vi "PROJEKAT RUKE-final.vi"() -> ()   [LabVIEW 2014]
doc: "This example shows a robotic arm with four revolute joints (a 4R serial robot), and demonstrates how to use custom equations to deterministically compute inverse kinematics for the arm."
uses:
  <vilib>/Analysis/Matrix/Datatypes/RealMatrix.ctl
  <vilib>/Platform/TimedLoop/XDataNode/timing_clust.ctl
  <vilib>/Platform/TimedLoop/XDataNode/nitl_modes.ctl
  <vilib>/Platform/TimedLoop/XDataNode/wakeup.ctl
  <vilib>/robotics/Kinematics/Plotting/Tree Element.ctl
  <vilib>/robotics/Kinematics/Plotting/Element Type.ctl
  <vilib>/robotics/Kinematics/Plotting/Joint Type.ctl
  Projekat SNJ+ED/Timer 2013/Control Timer.ctl
  <vilib>/Utility/inputDevices.llb/joystickAcquire.vi
  <vilib>/Analysis/Matrix/Numeric/Multiply/Multiply - R,RM.vi
  <vilib>/Analysis/Matrix/Numeric/Add/Add - RM,RM.vi
  <vilib>/Analysis/Matrix/Numeric/Multiply/Multiply - RM,R.vi
  <vilib>/NXT/Dual Mode Library/prims/inRangeAndCoerce/inRangeAndCoerce_float.vi
  <vilib>/addons/Fuzzy Logic/FL Fuzzy Controller (MISO).vi
  <vilib>/picture/3D Picture Control/Object/Create Object (name).vi
  <vilib>/picture/3D Picture Control/Helpers/Apply Texture (no reference).vi
  <vilib>/picture/3D Picture Control/Object/Add Object (no reference).vi
  <vilib>/Utility/inputDevices.llb/closeJoystick.vi
  <vilib>/platform/TimedLoop/XDataNode/XDataNode.xnode
  <vilib>/robotics/Kinematics/Plotting/NI_Robotics_3DKinematics.lvlib
  <vilib>/Analysis/Matrix/NI_Matrix.lvlib
  <vilib>/Platform/TimedLoop/XDataNode/XDNodeRunTimeDep.lvlib
  <vilib>/addons/Fuzzy Logic/NI_Fuzzy_Logic_API.lvlib
  <vilib>/picture/3D Picture Control/NI_3D Picture Control.lvlib
panel:
  in  "square":bool
  in  "Triangle":bool
  out "UDP Y":dbl(graph)
  out "UDP X":dbl(graph)
  out "UDP Y":dbl
  out "UDP X":dbl
  in  "Enum":T1(ring)
  out "output boosted":dbl
  out "fuzzy 1":dbl=-0.3643519039326156
  out "output":dbl=0.0001328998348474089
  in  "Kp2":dbl=120.0
  in  "Ki2":dbl=0.0005
  in  "Kd2":dbl=3.0
  in  "fuzzy za joint 2":bool=TRUE
  out "Fuzzy Kp":dbl=600.1063198678779
  in  "SMC J2":dbl=23.0
  in  "fuzzy za joint 1":bool=TRUE
  in  "Kp1":dbl=700.0
  out "Ycontroller":dbl
  out "Xcontroller":dbl
  in  "SMC J1":dbl=23.0
  in  "PID":bool=TRUE
  in  "stanja":T2
  in  "circle":bool
  in  "Kd1":dbl=20.0
  in  "Ki1":dbl=0.01
  out "error joint 2":dbl=0.8817520547054016
  out "error joint 1":dbl=-1.5374954740064481
  in  "Joint angles requested":dbl[](array[numeric])=[0.0, -2.3551534008356274, 2.0586714743351897, 0.0]
  out "Torque 2":sgl(graph)=9.405421
  out "Torque 1":sgl(graph)=-10.80559
  out "axis 2":cluster{"Joint Angles":dbl, "Joint Angles":dbl}(graph)={"Joint Angles"=117.07143482867573, "Joint Angles"=117.95318688338114}
  out "axis 1":cluster{"Joint Angles":dbl, "Joint Angles":dbl}(graph)={"Joint Angles"=-133.40285449975764, "Joint Angles"=-134.94034997376409}
  out "T requested":T3=[[-10.805589299068552], [9.40542142349445]]
  out "Qenc":T3=[[-2.3283250726964995], [2.0432778992607856]]
  out "dQenc":T3=[[-0.00014660765716752367], [-8.377580409572782e-05]]
  in  "enc resolution":dbl=900000.0
  out "dQ":T3=[[-0.0001628688682452542], [-6.482032013744222e-05]]
  out "Q":T3=[[-2.3283199705917617], [2.043281569449471]]
  out "T":T3=[[-10.80558967590332], [9.405421257019043]]
  in  "Y":dbl(slide)=-1.0 scale=-1.0..1.0
  in  "X":dbl(slide)=0.24999999999999994 scale=-1.5..1.5
  in  "actutator max torque":sgl(slide)=100.0 scale=0.0..100.0
  out "first overload":bool
  out "second overload":bool
  in  "controller on":bool=TRUE
  in  "Joint angles":dbl[](array[numeric])=[3.14, -2.3283199705917617, 2.043281569449471, 0.0]
  in  "stop":bool
  out "3D robotic arm":refnum<vi>(3d-picture)
  # "!!!VAZNO!!!\nPRE  POKRETANJA \n-POSTAVITI U TASK MANAGERU PRIORITET U REAL TIME\n-POKRENUTI PROJEKAT PA GA STOPIRATI I PONOVO POKRENUTI"
  # "Naèini kontrole"
  # "UDP za computer vision"
  # "HID uredjaj"
  # "Predefinisane putanje"
  # "Strategije upravljanja"
  # "PID parametri"
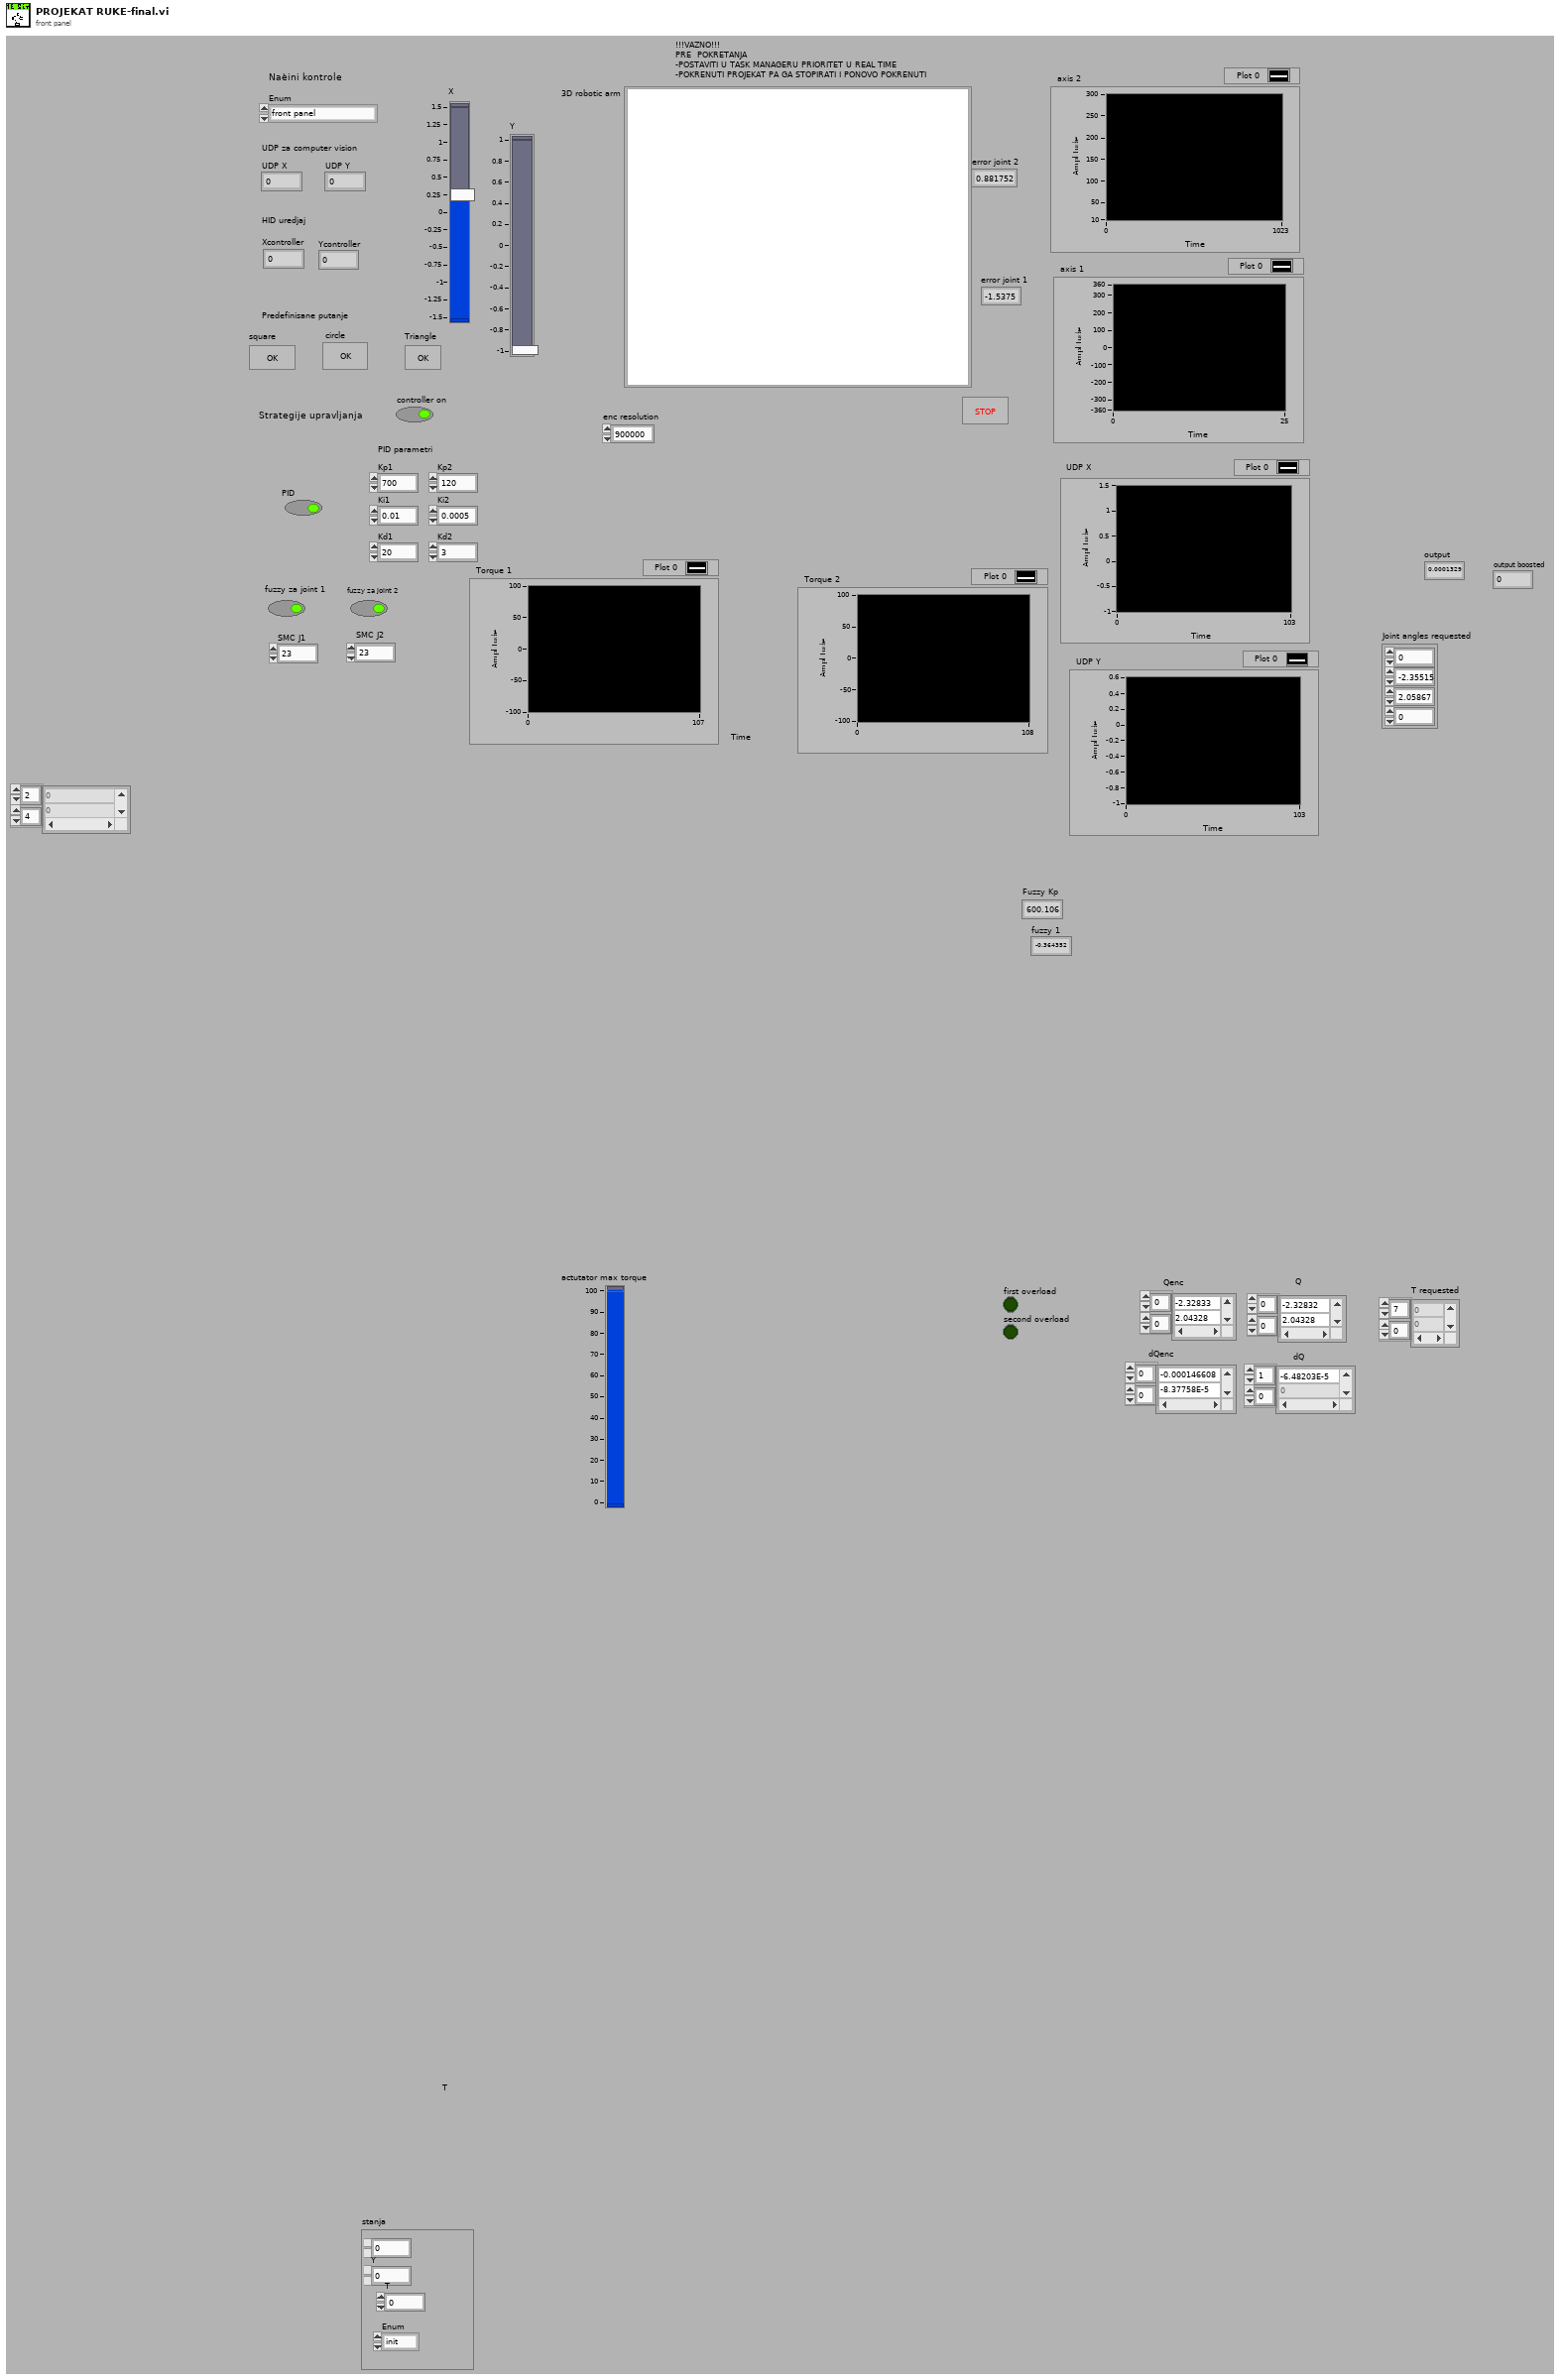
[diagram p1: front panel]
types:
  T1 = enum16{"front panel", "producer consumer", "hid", "udp"}
  T2 = cluster{"X":dbl, "Y":dbl, "T":dbl, "Enum":enum16{"init", "wait", "execute", "shutdown"}}
  T3 = typedef "NI_Matrix.lvlib/RealMatrix.ctl" = dbl[][]
  T4 = cluster{"Red":sgl, "Green":sgl, "Blue":sgl, "Alpha":sgl}
  T5 = typedef "NI_Robotics_3DKinematics.lvlib/Tree Element.ctl" = cluster{"Name":string, "Parent":string, "Type":T6, "Visible?":bool, "Geometry Definition":dbl[], "Position WRT Parent (X,Y,Z)":dbl[], "Rotation WRT Parent (degrees)":dbl[], "Joint Type":T7, "Geometry File Path":path, "Indent Level":i32, "Color":u32}
  T6 = typedef "NI_Robotics_3DKinematics.lvlib/Element Type.ctl" = enum16{"Joint", "Box", "Cylinder", "Cone", "Sphere", "ASE File", "VRML File", "STL File", "Space"}
  T7 = typedef "NI_Robotics_3DKinematics.lvlib/Joint Type.ctl" = enum16{"Trans_X", "Trans_Y", "Trans_Z", "Rot_X", "Rot_Y", "Rot_Z", "None"}
  T8 = typedef "NI_Fuzzy_Logic_API.lvlib/FL System.ctl" = cluster{"input variables":T9[], "output variables":T9[], "rules":T12[], "defuzzification method":T18, "description":string, "user MF interpolating polynomials":T19[]}
  T9 = typedef "NI_Fuzzy_Logic_API.lvlib/FL Variable.ctl" = cluster{"name":string, "range":dbl[], "MFs":T10[]}
  T10 = typedef "NI_Fuzzy_Logic_API.lvlib/FL Membership Function.ctl" = cluster{"name":string, "shape":T11, "points":dbl[], "color":u32, "user-defined shape index":i32}
  T11 = typedef "NI_Fuzzy_Logic_API.lvlib/FL Membership Function Shape.ctl" = u16
  T12 = typedef "NI_Fuzzy_Logic_API.lvlib/FL Rule.ctl" = cluster{"antecedents":T13[], "antecedent connective":T15, "consequents":T16[], "consequent implication":T17, "degree of support":dbl}
  T13 = typedef "NI_Fuzzy_Logic_API.lvlib/FL Antecedent.ctl" = cluster{"Var Index":i32, "MF Index":i32, "Cond":T14}
  T14 = typedef "NI_Fuzzy_Logic_API.lvlib/FL Modifier.ctl" = u16
  T15 = typedef "NI_Fuzzy_Logic_API.lvlib/FL Antecedent Connective.ctl" = u16
  T16 = typedef "NI_Fuzzy_Logic_API.lvlib/FL Consequent.ctl" = cluster{"Var Index":i32, "MF Index":i32, "Cond":T14}
  T17 = typedef "NI_Fuzzy_Logic_API.lvlib/FL Consequent Implication.ctl" = u16
  T18 = typedef "NI_Fuzzy_Logic_API.lvlib/FL Defuzzification.ctl" = u16
  T19 = typedef "NI_Fuzzy_Logic_API.lvlib/FL Interpolating polynomials.ctl" = cluster{"X":dbl[], "Y":dbl[], "Y(x) coeff":dbl[][], "X(y) coeff":dbl[][], "Area(y) coeff":dbl[][], "coa_x(y) coeff":dbl[][]}
  T20 = typedef "XDNodeRunTimeDep.lvlib/timing_clust.ctl" = cluster{"Expected End [f-1]":u64, "Actual End [f-1]":u64, "Finished Late? [f-1]":bool, "Expected End [i-1]":u64, "Actual End [i-1]":u64, "Finished Late? [i-1]":bool, "Expected Start [i]":u64, "Actual Start [i]":u64, "Expected Start [f]":u64, "Actual Start [f]":u64, "Source Name":string, "Structure Name":string, "Period":i64, "Deadline":i64, "Offset":i64, "Start":i64, "Priority":i32, "Timeout":i32, "Mode":T21, "Wakeup Reason":T22, "Error":errorcluster, "Source Type":string, "Secondary Source Type":string, "Global End Time":u64, "Global Start Time":u64, "Frame Duration":u64, "Iteration Duration":u64, "Assigned CPU":i32, "I/O Scan Engine Mode":u32}
  T21 = typedef "XDNodeRunTimeDep.lvlib/nitl_modes.ctl" = enum32{"No Change", "Process missed periods, maintain original phase", "Discard missed periods, maintain original phase", "Process missed periods, ignore original phase", "Discard missed periods, ignore original phase"}
  T22 = typedef "XDNodeRunTimeDep.lvlib/wakeup.ctl" = enum32{"Normal", "Aborted", "Asynchronous wakeup", "Timing source error", "Timed loop error", "Timeout"}
  T23 = typedef "NI_Robotics_3DKinematics.lvlib/Joint Control.ctl" = cluster{"Joint Refnum":refnum<vi>, "Joint Type":T7, "Position WRT Parent":dbl[], "Rotation WRT Parent":dbl[], "Bar Refnum":refnum<vi>}
  T24 = typedef "Control Timer.ctl" = enum16{"Timecheck", "Reset"}
  T25 = typedef "imagedata.ctl" = cluster{"image type":i32, "image depth":i32, "image":u8[], "mask":u8[], "colors":u32[], "Rectangle":cluster{"left":i16, "top":i16, "right":i16, "bottom":i16}}
  T26 = cluster{"X":dbl, "Y":dbl, "T":dbl, "Enum":enum16{"init", "wait", "execute", "shutdown"}}[]
  T27 = cluster{"X axis":i32, "Y axis":i32, "Z axis":i32, "X axis rotation":i32, "Y axis rotation":i32, "Z axis rotation":i32, "U axis":i32, "V axis":i32}
  T28 = cluster{"button 1":bool, "button 2":bool, "button 3":bool, "button 4":bool, "button 5":bool, "button 6":bool, "button 7":bool, "button 8":bool, "button 9":bool, "button 10":bool, "button 11":bool, "button 12":bool, "button 13":bool, "button 14":bool, "button 15":bool, "button 16":bool, "button 17":bool, "button 18":bool, "button 19":bool, "button 20":bool, "button 21":bool, "button 22":bool, "button 23":bool, "button 24":bool, "button 25":bool, "button 26":bool, "button 27":bool, "button 28":bool, "button 29":bool, "button 30":bool, "button 31":bool, "button 32":bool}
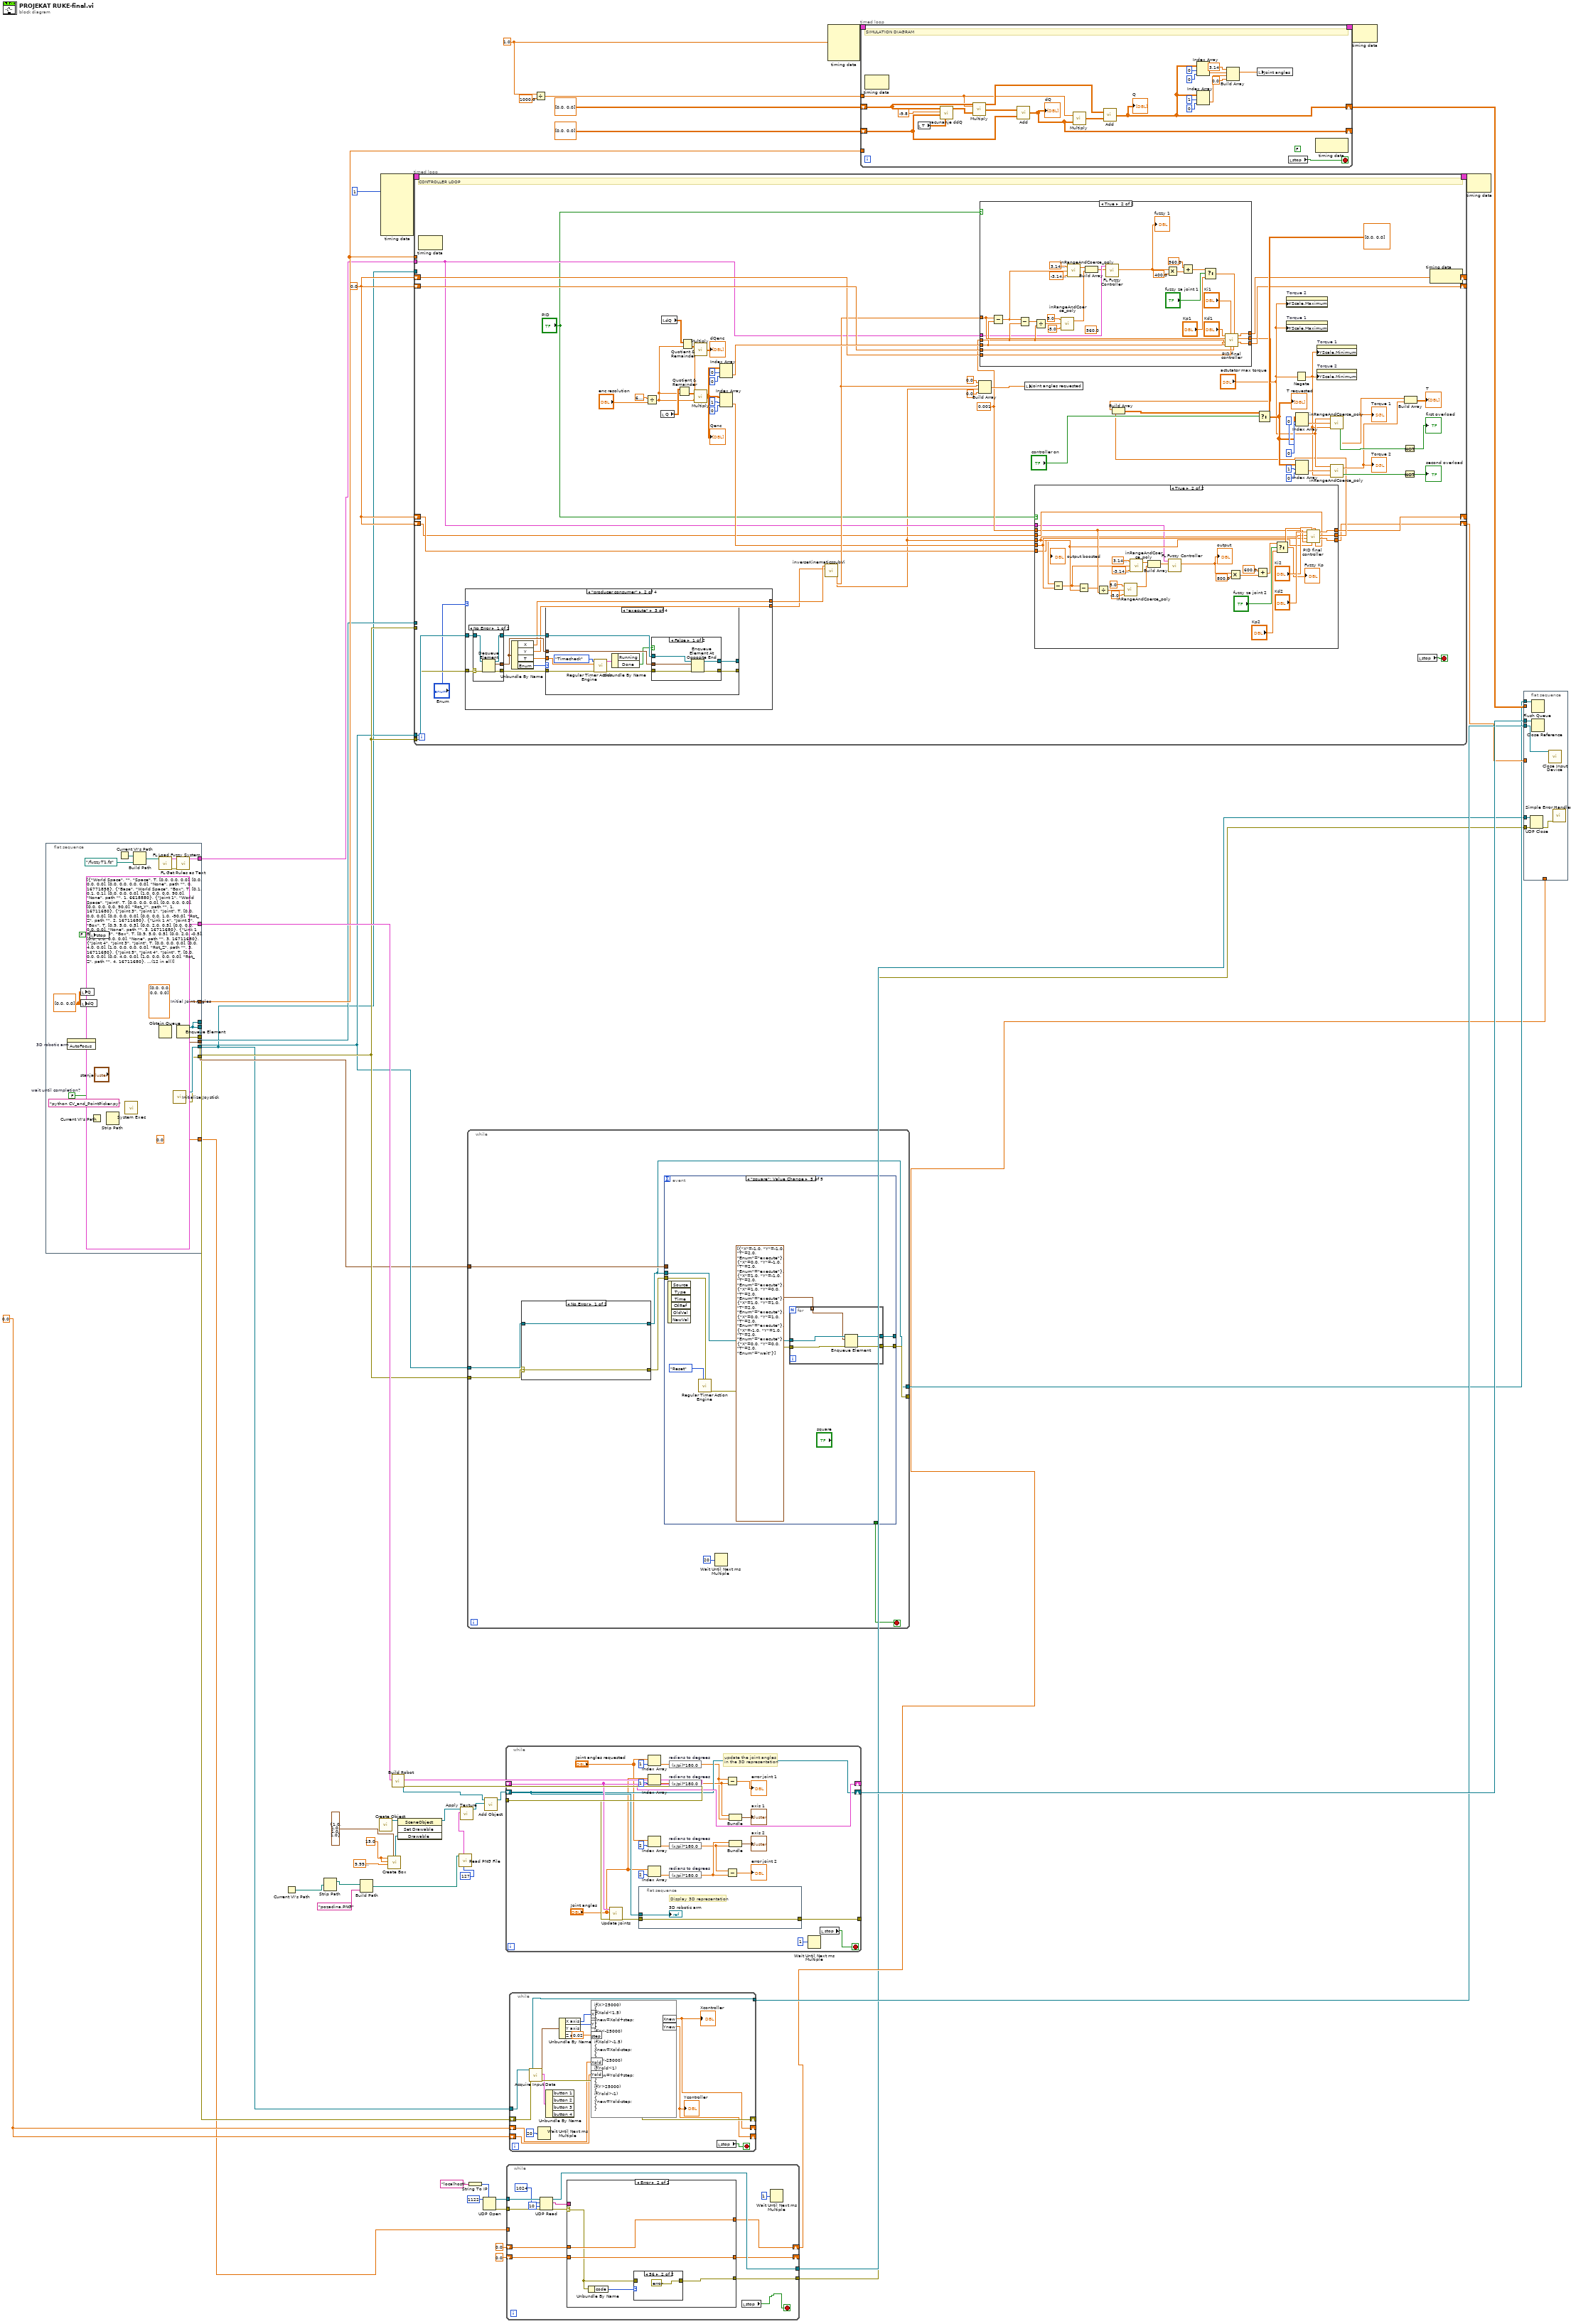
[diagram p0: block diagram]
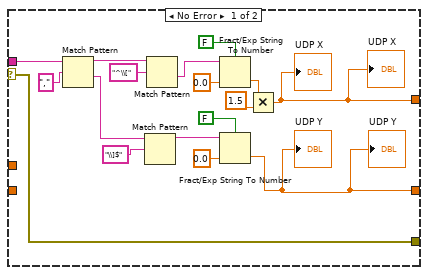
[diagram p2: hidden frame]
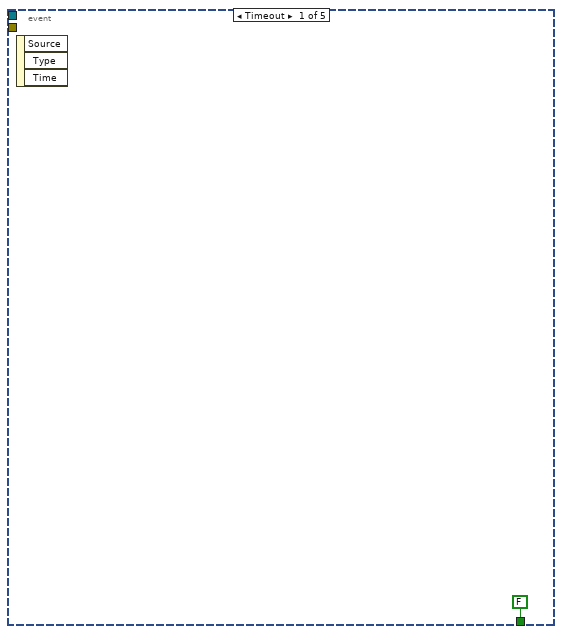
[diagram p4: hidden frame]
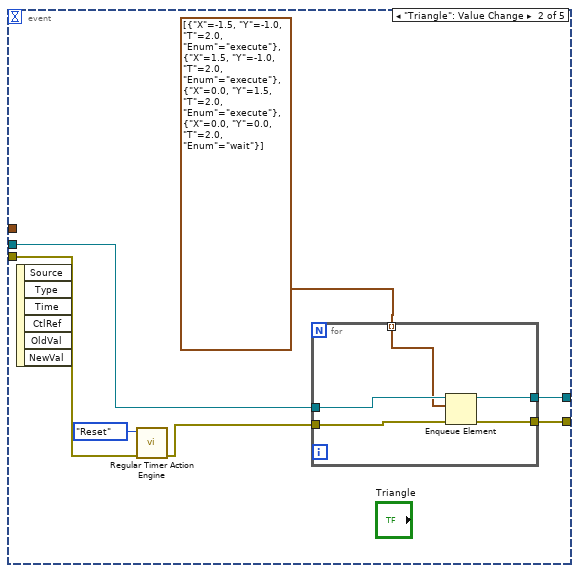
[diagram p5: hidden frame]
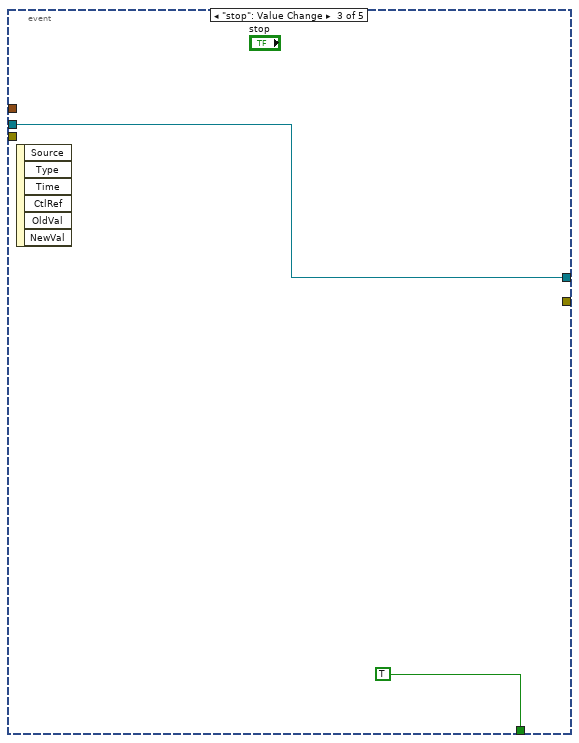
[diagram p6: hidden frame]
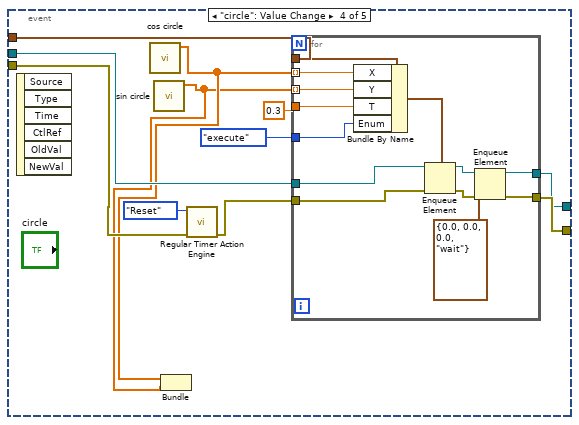
[diagram p7: hidden frame]
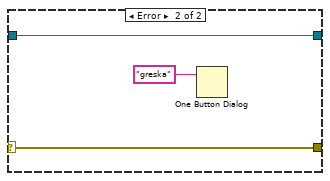
[diagram p8: hidden frame]
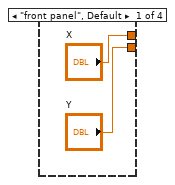
[diagram p9: hidden frame]
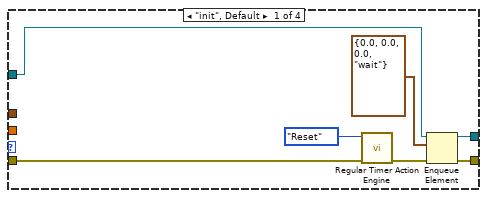
[diagram p10: hidden frame]
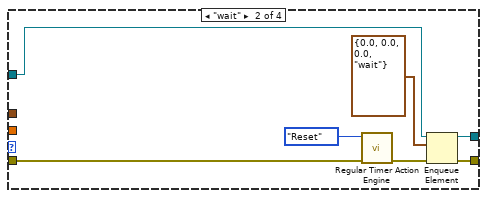
[diagram p11: hidden frame]
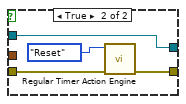
[diagram p12: hidden frame]
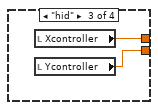
[diagram p15: hidden frame]
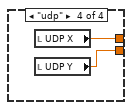
[diagram p16: hidden frame]
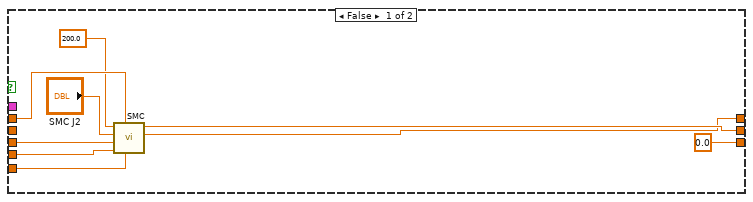
[diagram p17: hidden frame]
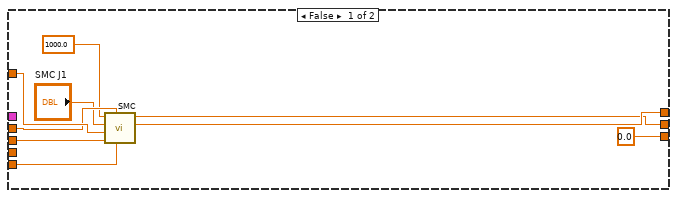
[diagram p18: hidden frame]
diagram:
  w23 = 0.0
  w26 = sgl 15.0 ("Length X")
  w38 = 0.0
  w39 = 1.0 ("simulation precision")
  n1 = flat-sequence {
    tunnel: [w76] -> w42
    tunnel: [T5[] [{"Name"="World Space", "Parent"="", "Type"=enum."Space", "Visible?"=TRUE, "Geometry Definition"=[0.0, 0.0, 0.0], "Position WRT Parent (X,Y,Z)"=[0.0, 0.0, 0.0], "Rotation WRT Parent (degrees)"=[0.0, 0.0, 0.0, 0.0], "Joint Type"=enum."None", "Geometry File Path"=path "", "Indent Level"=0, "Color"=16771858}, {"Name"="Base", "Parent"="World Space", "Type"=enum."Box", "Visible?"=TRUE, "Geometry Definition"=[0.1, 0.1, 0.1], "Position WRT Parent (X,Y,Z)"=[0.0, 0.0, 0.0], "Rotation WRT Parent (degrees)"=[1.0, 0.0, 0.0, 90.0], "Joint Type"=enum."None", "Geometry File Path"=path "", "Indent Level"=1, "Color"=6618880}, {"Name"="Joint 1", "Parent"="World Space", "Type"=enum."Joint", "Visible?"=TRUE, "Geometry Definition"=[0.0, 0.0, 0.0], "Position WRT Parent (X,Y,Z)"=[0.0, 0.0, 0.0], "Rotation WRT Parent (degrees)"=[0.0, 0.0, 0.0, 90.0], "Joint Type"=enum."Rot_Y", "Geometry File Path"=path "", "Indent Level"=1, "Color"=16711680}, {"Name"="Joint 3", "Parent"="Joint 1", "Type"=enum."Joint", "Visible?"=TRUE, "Geometry Definition"=[0.0, 0.0, 0.0], "Position WRT Parent (X,Y,Z)"=[0.0, 0.0, 0.0], "Rotation WRT Parent (degrees)"=[0.0, 0.0, 1.0, -90.0], "Joint Type"=enum."Rot_Z", "Geometry File Path"=path "", "Indent Level"=2, "Color"=16711680}, {"Name"="Link 1 A", "Parent"="Joint 3", "Type"=enum."Box", "Visible?"=TRUE, "Geometry Definition"=[0.9, 5.0, 0.5], "Position WRT Parent (X,Y,Z)"=[0.0, 2.0, 0.5], "Rotation WRT Parent (degrees)"=[0.0, 0.0, 0.0, 0.0], "Joint Type"=enum."None", "Geometry File Path"=path "", "Indent Level"=3, "Color"=16711680}, {"Name"="Link 1 B", "Parent"="Joint 3", "Type"=enum."Box", "Visible?"=TRUE, "Geometry Definition"=[0.9, 5.0, 0.5], "Position WRT Parent (X,Y,Z)"=[0.0, 2.0, -0.5], "Rotation WRT Parent (degrees)"=[0.0, 0.0, 0.0, 0.0], "Joint Type"=enum."None", "Geometry File Path"=path "", "Indent Level"=3, "Color"=16711680}, {"Name"="Joint 4", "Parent"="Joint 3", "Type"=enum."Joint", "Visible?"=TRUE, "Geometry Definition"=[0.0, 0.0, 0.0], "Position WRT Parent (X,Y,Z)"=[0.0, 4.0, 0.0], "Rotation WRT Parent (degrees)"=[1.0, 0.0, 0.0, 0.0], "Joint Type"=enum."Rot_Z", "Geometry File Path"=path "", "Indent Level"=3, "Color"=16711680}, {"Name"="Joint 5", "Parent"="Joint 4", "Type"=enum."Joint", "Visible?"=TRUE, "Geometry Definition"=[0.0, 0.0, 0.0], "Position WRT Parent (X,Y,Z)"=[0.0, 4.0, 0.0], "Rotation WRT Parent (degrees)"=[1.0, 0.0, 0.0, 0.0], "Joint Type"=enum."Rot_Z", "Geometry File Path"=path "", "Indent Level"=4, "Color"=16711680}, {"Name"="Lower Arm 1", "Parent"="Joint 4", "Type"=enum."Box", "Visible?"=TRUE, "Geometry Definition"=[0.9, 4.5, 0.5], "Position WRT Parent (X,Y,Z)"=[0.0, 1.75, 0.5], "Rotation WRT Parent (degrees)"=[0.0, 0.0, 0.0, 0.0], "Joint Type"=enum."None", "Geometry File Path"=path "", "Indent Level"=5, "Color"=16860}, {"Name"="Lower Arm 2", "Parent"="Joint 4", "Type"=enum."Box", "Visible?"=TRUE, "Geometry Definition"=[0.9, 4.5, 0.5], "Position WRT Parent (X,Y,Z)"=[0.0, 1.75, -0.5], "Rotation WRT Parent (degrees)"=[0.0, 0.0, 0.0, 0.0], "Joint Type"=enum."None", "Geometry File Path"=path "", "Indent Level"=5, "Color"=16860}, {"Name"="Hand", "Parent"="Joint 4", "Type"=enum."Box", "Visible?"=TRUE, "Geometry Definition"=[1.0, 0.375, 1.0], "Position WRT Parent (X,Y,Z)"=[0.0, 4.0, 0.0], "Rotation WRT Parent (degrees)"=[0.0, 1.0, 0.0, 0.0], "Joint Type"=enum."None", "Geometry File Path"=path "", "Indent Level"=5, "Color"=16711680}, {"Name"="TCF", "Parent"="Joint 4", "Type"=enum."Cylinder", "Visible?"=TRUE, "Geometry Definition"=[0.4, 0.2, 0.1], "Position WRT Parent (X,Y,Z)"=[0.0, 4.5, 0.0], "Rotation WRT Parent (degrees)"=[1.0, 0.0, 0.0, 90.0], "Joint Type"=enum."None", "Geometry File Path"=path "", "Indent Level"=5, "Color"=16776960}]] -> w51
    tunnel: [w73] -> w25
    tunnel: [w72] -> w24
    tunnel: [w66] -> w37
    tunnel: [w63] -> w35
    tunnel: [w62] -> w36
    tunnel: [w62] -> w34
    tunnel: ["stanja"] -> w33
    tunnel: [0.0] -> w1
    frame #0 {
      w60 = FALSE  # wait until completion?
      w74 = T3 [[0.0], [0.0]] ("Q")
      w76 = dbl[] [0.0, 0.0, 0.0, 0.0]  # Initial Joint Angles
      n2 = invoke on="3D robotic arm" class="SceneGraphDisp (strict)" method="AutoFocus"() -> ()  [unwired: 3 in, 3 out]
      n3 = local write "Q"(w74) -> ()
      n4 = local write "dQ"(w74) -> ()
      n5 = local write "stop"(FALSE ("stop")) -> ()
      n6 = Current VI's Path() -> (path=w58:path)
      n7 = Strip Path(path=w58) -> (stripped path=w57:path)  [unwired: 1 out]
      n8 = Current VI's Path() -> (path=w69:path)
      n9 = call <vilib>:"System Exec.vi"("wait until completion? (T)"=w60, "working directory"=w57, "command line"="python CV_and_PointPicker.py") -> ()  [unwired: 3 in, 6 out]
      n10 = Build Path(base path=w69, name or relative path=path "../fuzzyT1.fs") -> (appended path=w70:path)
      n11 = call <vilib>:"FL Load Fuzzy System.vi"("file path"=w70) -> ("error out"=w67:errorcluster, "fuzzy system out"=w68:T8)  [unwired: 1 in, 8 out]
      n12 = Obtain Queue(element data type="stanja") -> (queue out=w64:refnum<queue>, error out=w65:errorcluster)  [unwired: 4 in, 1 out]
      n13 = call <vilib>:"Initialize Joystick.vi"() -> ("error out"=w72:errorcluster, "device ID"=w73:refnum<k1>)  [unwired: 10 in]
      n14 = call <vilib>:"FL Get Rules as Text.vi"("error in (no error)"=w67, "fuzzy system in"=w68) -> ("fuzzy system out"=w66:T8)  [unwired: 7 in, 2 out]
      n15 = Enqueue Element(queue=w64, element="stanja", error in (no error)=w65) -> (queue out=w62:refnum<queue>, error out=w63:errorcluster)  [unwired: 1 in, 1 out]
    }
  }
  n16 = Current VI's Path() -> (path=w7:path)
  n17 = Strip Path(path=w7) -> (stripped path=w6:path)  [unwired: 1 out]
  n18 = Build Path(base path=w6, name or relative path="pozadina.PNG") -> (appended path=w8:path)
  n19 = call-poly <vilib>:"Create Object.vi"() -> ("Scene:New Object"=w32:refnum<vi>)  [unwired: 10 in, 1 out]
  n20 = node-c288(i64 1 ("Period")) -> (w46:T20)  [unwired: 7 in]
  n21 = call <vilib>:"Create Box.vi"("Color"=T4 {"Red"=1.0, "Green"=1.0, "Blue"=1.0, "Alpha"=1.0}, "Length Z"=sgl 0.0001, "Length Y"=w26, "Length X"=w26) -> ("New Box Refnum"=w31:refnum<vi>)  [unwired: 6 in, 1 out]
  n22 = call <vilib>:"Build Robot.vi"("Robot Elements"=w51) -> ("error out"=w52:errorcluster, "Scene Out"=w29:refnum<vi>, "Joint Array"=w53:T23[])  [unwired: 8 in]
  n23 = invoke class="SceneObject" method="Set Drawable"(reference=w32, "Drawable"=w31) -> (reference out=w22:refnum<vi>)  [unwired: 2 in, 3 out]
  n24 = timed-loop "e" {
    timing: w46 -> [_]
    timing-out: [_] -> w45
    tunnel: w42 -> [_]
    tunnel: w25 -> [_]
    shift-right: [w100] -> _
    shift-left: w38 -> [w97]
    shift-right: [w83] -> w10
    shift-left: w38 -> [w88]
    shift-right: [w99] -> _
    shift-left: w38 -> [w96]
    shift-right: [w84] -> _
    shift-left: w38 -> [w89]
    tunnel: w37 -> [w87]
    tunnel: w35 -> [_]
    tunnel: w36 -> [_]
    tunnel: w35 -> [w81]
    tunnel: w34 -> [w82]
    stop <- w134 stop-if-true
    w90 = 0.001 ("Ts")
    # "CONTROLLER LOOP"
    n25 = node-c288() -> ()  [unwired: 1 in, 1 out]
    n26 = case shown="\"producer consumer\"" "Enum" {
      tunnel: ["X" w138 w189 w191] -> w80
      tunnel: ["Y" w137 w188 w190] -> w79
      tunnel: w82 -> [_ w140 _ _]
      tunnel: w81 -> [_ w139 _ _]
      frame "front panel", Default {
      }
      frame "producer consumer" {
        n27 = case shown="No Error" w139 {
          selector: w139 -> [w181 w186]
          tunnel: [w182 w186] -> w141
          tunnel: w140 -> [w185 w187]
          tunnel: [w184 w187] -> w142
          tunnel: [w183 _] -> w143
          frame No Error {
            n28 = Dequeue Element(queue=w185, error in (no error)=w181) -> (queue out=w184:refnum<queue>, element=w183:T2, error out=w182:errorcluster)  [unwired: 1 in, 1 out]
          }
          frame Error {
          }
        }
        n29 = Unbundle By Name(w143) -> ("X"=w138:dbl, "Y"=w137:dbl, "T"=w144:dbl, "Enum"=w145:enum16{"init", "wait", "execute", "shutdown"})
        n30 = case shown="\"execute\"" w145 {
          tunnel: w141 -> [w147 w155 w169 w179]
          tunnel: w142 -> [w152 w156 w166 w180]
          tunnel: w143 -> [_ _ w165 _]
          tunnel: w144 -> [_ _ w164 _]
          tunnel: [w150 w153 w160 w180] -> _
          tunnel: [w149 w154 w161 w179] -> _
          frame "init", Default {
            n31 = call "Regular Timer Action Engine.vi"("Enum"=Control_Timer."Reset", "error in"=w147) -> ("error out"=w146:errorcluster)  [unwired: 7 in, 1 out]
            n32 = Enqueue Element(queue=w152, element=T2 {"X"=0.0, "Y"=0.0, "T"=0.0, "Enum"=enum."wait"}, error in (no error)=w146) -> (queue out=w150:refnum<queue>, error out=w149:errorcluster)  [unwired: 1 in, 1 out]
          }
          frame "wait" {
            n33 = call "Regular Timer Action Engine.vi"("Enum"=Control_Timer."Reset", "error in"=w155) -> ("error out"=w157:errorcluster)  [unwired: 7 in, 1 out]
            n34 = Enqueue Element(queue=w156, element=T2 {"X"=0.0, "Y"=0.0, "T"=0.0, "Enum"=enum."wait"}, error in (no error)=w157) -> (queue out=w153:refnum<queue>, error out=w154:errorcluster)  [unwired: 1 in, 1 out]
          }
          frame "execute" {
            n35 = call "Regular Timer Action Engine.vi"("Enum"=Control_Timer."Timecheck", "Time Target"=w164, "error in"=w169) -> ("Status"=w168:cluster{"Running":bool, "Done":bool}, "error out"=w167:errorcluster)  [unwired: 6 in]
            n36 = Unbundle By Name(w168) -> ("Done"=w163:bool)  [unwired: 1 out]
            n37 = case shown="False" w163 {
              tunnel: w167 -> [w173 w177]
              tunnel: w166 -> [w174 w175]
              tunnel: [w172 w176] -> w161
              tunnel: w165 -> [w171 _]
              tunnel: [w170 w175] -> w160
              frame False {
                n38 = Enqueue Element At Opposite End(queue=w174, element=w171, error in (no error)=w173) -> (queue out=w170:refnum<queue>, error out=w172:errorcluster)  [unwired: 1 in, 1 out]
              }
              frame True {
                n39 = call "Regular Timer Action Engine.vi"("Enum"=Control_Timer."Reset", "error in"=w177) -> ("error out"=w176:errorcluster)  [unwired: 7 in, 1 out]
              }
            }
          }
          frame "shutdown" {
          }
        }
      }
      frame "hid" {
        n40 = local read "Xcontroller"() -> (w189:dbl)
        n41 = local read "Ycontroller"() -> (w188:dbl)
      }
      frame "udp" {
        n42 = local read "UDP X"() -> (w191:dbl)
        n43 = local read "UDP Y"() -> (w190:dbl)
      }
    }
    n44 = Divide(x=6.283185307179586, y="enc resolution") -> (x/y=w119:dbl)
    n45 = local read "Q"() -> (w122:T3)
    n46 = local read "dQ"() -> (w118:T3)
    n47 = Quotient & Remainder(x=w122, y=w119) -> (floor(x/y)=w121:T3)  [unwired: 1 out]
    n48 = Quotient & Remainder(x=w118, y=w119) -> (floor(x/y)=w120:T3)  [unwired: 1 out]
    n49 = call-poly <vilib>:"Multiply.vi"("Real Scalar c"=w119, "Real Matrix A"=w120) -> ("A * c"=→"dQenc":T3)
    n50 = call-poly <vilib>:"Multiply.vi"("Real Scalar c"=w119, "Real Matrix A"=w121) -> ("A * c"=w94:T3)
    "Qenc" <- w94
    n51 = Index Array(array=w94, index (row)=0, index (col)=0) -> (element=w101:dbl)
    n52 = Index Array(array=w94, index (row)=1, index (col)=0) -> (element=w91:dbl)
    n53 = call "inverseKinematicssubVi.vi"("y"=w79, "x"=w80) -> ("second joint"=w78:dbl, "first joint"=w95:dbl)  [unwired: 8 in]
    n54 = Build Array(0.0 ("element"), w95, w78, 0.0 ("element")) -> (w106:dbl[])
    n55 = case shown="True" "PID" {
      tunnel: w101 -> [w237 w254]
      tunnel: [0.0 ("sum_out") w267] -> w100
      tunnel: [w234 w266] -> w99
      tunnel: [w233 w265] -> w98
      tunnel: w97 -> [_ w264]
      tunnel: w96 -> [w236 w261]
      tunnel: w95 -> [w238 w255]
      tunnel: w90 -> [w235 w252]
      tunnel: w87 -> [_ w250]
      frame False {
        n56 = call "SMC.vi"("e_prev"=w236, "t"=w235, "q"=w237, "SP"=w238, "a"="SMC J1", "gain"=1000.0) -> ("e_out"=w234:dbl, "u"=w233:dbl)  [unwired: 4 in]
      }
      frame True {
        (unwired) 560.0 ("x")
        n57 = Subtract(x=w255, y=w254) -> (x-y=w248:dbl)
        n58 = Subtract(x=w248, y=w252) -> (x-y=w251:dbl)
        n59 = Divide(x=w251, y=w252) -> (x/y=w247:dbl)
        n60 = call-poly <vilib>:"inRangeAndCoerce_poly.vi"("lower limit"=sgl -5.0 ("upper limit"), "x"=w247, "upper limit"=sgl 5.0) -> ("coerced(x)"=w245:sgl)  [unwired: 1 out]
        n61 = call-poly <vilib>:"inRangeAndCoerce_poly.vi"("lower limit"=sgl -3.14, "x"=w248, "upper limit"=sgl 3.14) -> ("coerced(x)"=w246:sgl)  [unwired: 1 out]
        n62 = Build Array(w246, w245) -> (w249:sgl[])
        n63 = call-poly <vilib>:"FL Fuzzy Controller.vi"("input values"=w249, "fuzzy system in"=w250) -> ("output value"=w260:dbl)  [unwired: 1 in, 8 out]
        "fuzzy 1" <- w260
        n64 = Multiply(x=w260, y=400.0) -> (x*y=w257:dbl)
        n65 = Add(x=560.0, y=w257) -> (x+y=w256:dbl)
        n66 = Select(t=w256, s="fuzzy za joint 1", f="Kp1") -> (s? t:f=w240:dbl)
        n67 = call "PID final controller.vi"("e_sum"=w264, "Kp"=w240, "e_t"=w261, "Ki"="Ki1", "Ts"=w252, "q"=w254, "SP"=w255, "Kd"="Kd1") -> ("sum_out"=w267:dbl, "u_out"=w265:dbl, "e_out"=w266:dbl)  [unwired: 1 in]
      }
    }
    n68 = local write "Joint angles requested"(w106) -> ()
    n69 = case shown="True" "PID" {
      tunnel: w91 -> [w200 w215]
      tunnel: [0.0 ("sum_out") w229] -> w83
      tunnel: [w196 w228] -> w84
      tunnel: [w197 w227] -> w85
      tunnel: w89 -> [w198 w214]
      tunnel: w90 -> [w199 w216]
      tunnel: w88 -> [_ w224]
      tunnel: w87 -> [_ w212]
      tunnel: w78 -> [w192 w201]
      frame False {
        n70 = call "SMC.vi"("e_prev"=w198, "t"=w199, "q"=w200, "SP"=w192, "a"="SMC J2", "gain"=200.0) -> ("e_out"=w196:dbl, "u"=w197:dbl)  [unwired: 4 in]
      }
      frame True {
        n71 = Subtract(x=w201, y=w215) -> (x-y=w207:dbl)
        n72 = Subtract(x=w207, y=w214) -> (x-y=w213:dbl)
        n73 = Divide(x=w213, y=w216) -> (x/y=w205:dbl)
        n74 = call-poly <vilib>:"inRangeAndCoerce_poly.vi"("lower limit"=sgl -5.0 ("upper limit"), "x"=w205, "upper limit"=sgl 5.0) -> ("coerced(x)"=w202:sgl)  [unwired: 1 out]
        n75 = call-poly <vilib>:"inRangeAndCoerce_poly.vi"("lower limit"=sgl -3.14, "x"=w207, "upper limit"=sgl 3.14) -> ("coerced(x)"=w206:sgl)  [unwired: 1 out]
        n76 = Build Array(w206, w202) -> (w217:sgl[])
        n77 = call-poly <vilib>:"FL Fuzzy Controller.vi"("input values"=w217, "fuzzy system in"=w212) -> ("output value"=w211:dbl)  [unwired: 1 in, 8 out]
        "output" <- w211
        n78 = Multiply(x=w211, y=800.0) -> (x*y=w210:dbl)
        n79 = Add(x=600.0, y=w210) -> (x+y=w223:dbl)
        n80 = Select(t=w223, s="fuzzy za joint 2", f="Kp2") -> (s? t:f=w220:dbl)
        "Fuzzy Kp" <- w220
        n81 = call "PID final controller.vi"("e_sum"=w224, "Kp"=w220, "e_t"=w214, "Ki"="Ki2", "Ts"=w216, "q"=w215, "SP"=w201, "Kd"="Kd2") -> ("sum_out"=w229:dbl, "u_out"=w227:dbl, "e_out"=w228:dbl)  [unwired: 1 in]
      }
    }
    n82 = Build Array(w98, w85) -> (w92:T3)
    n83 = Select(t=w92, s="controller on", f=T3 [[0.0], [0.0]]) -> (s? t:f=w129:T3)
    "T requested" <- w129
    n84 = property on="Torque 2" class="WFChart (strict)"("YScale.Maximum"="actutator max torque") -> ()  [unwired: 2 in, 2 out]
    n85 = property on="Torque 1" class="WFChart (strict)"("YScale.Maximum"="actutator max torque") -> ()  [unwired: 2 in, 2 out]
    n86 = Negate(x="actutator max torque") -> (-x=w109:sgl)
    n87 = Index Array(array=w129, index (row)=0, index (col)=0) -> (element=w128:dbl)
    n88 = Index Array(array=w129, index (row)=1, index (col)=0) -> (element=w126:dbl)
    n89 = property on="Torque 1" class="WFChart (strict)"("YScale.Minimum"=w109) -> ()  [unwired: 2 in, 2 out]
    n90 = property on="Torque 2" class="WFChart (strict)"("YScale.Minimum"=w109) -> ()  [unwired: 2 in, 2 out]
    n91 = call-poly <vilib>:"inRangeAndCoerce_poly.vi"("lower limit"=w109, "x"=w128, "upper limit"="actutator max torque") -> ("In Range?"=w115:bool, "coerced(x)"=w112:sgl)
    "Torque 1" <- w112
    n92 = call-poly <vilib>:"inRangeAndCoerce_poly.vi"("lower limit"=w109, "x"=w126, "upper limit"="actutator max torque") -> ("In Range?"=w117:bool, "coerced(x)"=w111:sgl)
    "Torque 2" <- w111
    n93 = Not(x=w115) -> (.not. x?=→"first overload":bool)
    n94 = Not(x=w117) -> (.not. x?=→"second overload":bool)
    n95 = Build Array(w112, w111) -> (→"T":T3)
    n96 = local read "stop"() -> (w134:bool)
    n97 = node-c288() -> ()  [unwired: 1 in, 1 out]
  }
  n98 = call <vilib>:"Read PNG File.vi"("Transparency Thresh"=u8 127, "path to PNG file"=w8) -> ("image data"=w20:T25)  [unwired: 7 in, 2 out]
  n99 = call-poly <vilib>:"Apply Texture.vi"("Image Data"=w20, "Scene Object In"=w22) -> ("Scene Object Out"=w21:refnum<vi>)  [unwired: 8 in, 1 out]
  n100 = while {
    tunnel: w35 -> [w277]
    tunnel: w34 -> [w276]
    tunnel: [w275] -> _
    tunnel: [w270] -> w5
    tunnel: w33 -> [w274]
    stop <- w272 stop-if-true
    n101 = case shown="No Error" w277 {
      selector: w277 -> [w330 w333]
      tunnel: [w330 w333] -> w273
      tunnel: w276 -> [w329 w332]
      tunnel: [w329 w332] -> w270
      frame No Error {
      }
      frame Error {
        n102 = One Button Dialog(message="greska") -> ()  [unwired: 1 in, 1 out]
      }
    }
    n103 = event shown="[4] \"square\": Value Change" {
      selector: _ -> [_ _ _ _ _]
      dyn-events: _ -> [_ _ _ _ _]
      timeout: _ -> [_ _ _ _ _]
      tunnel: w273 -> [_ w282 _ w300 w320]
      tunnel: w270 -> [_ w285 w291 w303 w323]
      tunnel: [_ w284 _ w302 w322] -> w275
      tunnel: [_ w283 w291 w301 w321] -> _
      tunnel: w274 -> [_ _ _ w297 _]
      tunnel: [FALSE _ TRUE _ _] -> w272
      event Timeout {
        n104 = event-data() -> ()  [unwired: 1 in, 3 out]
      }
      event "Triangle": Value Change {
        n105 = event-data() -> ()  [unwired: 1 in, 6 out]
        n106 = call "Regular Timer Action Engine.vi"("Enum"=Control_Timer."Reset", "error in"=w282) -> ("error out"=w281:errorcluster)  [unwired: 7 in, 1 out]
        n107 = for {
          tunnel: w281 -> [w289]
          tunnel: w285 -> [w290]
          tunnel: [w288] -> w284
          tunnel: [w287] -> w283
          tunnel: T26 [{"X"=-1.5, "Y"=-1.0, "T"=2.0, "Enum"=enum."execute"}, {"X"=1.5, "Y"=-1.0, "T"=2.0, "Enum"=enum."execute"}, {"X"=0.0, "Y"=1.5, "T"=2.0, "Enum"=enum."execute"}, {"X"=0.0, "Y"=0.0, "T"=2.0, "Enum"=enum."wait"}] -> [w286] mode=indexing
          n108 = Enqueue Element(queue=w290, element=w286, error in (no error)=w289) -> (queue out=w287:refnum<queue>, error out=w288:errorcluster)  [unwired: 1 in, 1 out]
        }
      }
      event "stop": Value Change {
        n109 = event-data() -> ()  [unwired: 1 in, 6 out]
      }
      event "circle": Value Change {
        n110 = event-data() -> ()  [unwired: 1 in, 6 out]
        n111 = call "cos circle.vi"() -> ("cos(x)"=w294:dbl[])  [unwired: 11 in]
        n112 = call "sin circle.vi"() -> ("sin(x)"=w293:dbl[])  [unwired: 11 in]
        n113 = Bundle("cos(x)"=w294, "sin(x)"=w293) -> ()  [unwired: 1 in, 1 out]
        n114 = call "Regular Timer Action Engine.vi"("Enum"=Control_Timer."Reset", "error in"=w300) -> ("error out"=w299:errorcluster)  [unwired: 7 in, 1 out]
        n115 = for {
          tunnel: w299 -> [w315]
          tunnel: w303 -> [w316]
          tunnel: [w307] -> w302
          tunnel: [w305] -> w301
          tunnel: w294 -> [w313] mode=indexing
          tunnel: w297 -> [w312]
          tunnel: w293 -> [w311] mode=indexing
          tunnel: 0.3 ("T") -> [w310]
          tunnel: enum16{"init", "wait", "execute", "shutdown"}."execute" ("Enum") -> [w309]
          n116 = Bundle By Name(cluster=w312, "X"=w313, "Y"=w311, "T"=w310, "Enum"=w309) -> (w314:T2)
          n117 = Enqueue Element(queue=w316, element=w314, error in (no error)=w315) -> (queue out=w306:refnum<queue>, error out=w308:errorcluster)  [unwired: 1 in, 1 out]
          n118 = Enqueue Element(queue=w306, element=T2 {"X"=0.0, "Y"=0.0, "T"=0.0, "Enum"=enum."wait"}, error in (no error)=w308) -> (queue out=w305:refnum<queue>, error out=w307:errorcluster)  [unwired: 1 in, 1 out]
        }
      }
      event "square": Value Change {
        n119 = event-data() -> ()  [unwired: 1 in, 6 out]
        n120 = call "Regular Timer Action Engine.vi"("Enum"=Control_Timer."Reset", "error in"=w320) -> ("error out"=w319:errorcluster)  [unwired: 7 in, 1 out]
        n121 = for {
          tunnel: w319 -> [w327]
          tunnel: w323 -> [w328]
          tunnel: [w326] -> w322
          tunnel: [w325] -> w321
          tunnel: T26 [{"X"=-1.0, "Y"=-1.0, "T"=2.0, "Enum"=enum."execute"}, {"X"=0.0, "Y"=-1.0, "T"=2.0, "Enum"=enum."execute"}, {"X"=1.0, "Y"=-1.0, "T"=2.0, "Enum"=enum."execute"}, {"X"=1.0, "Y"=0.0, "T"=2.0, "Enum"=enum."execute"}, {"X"=1.0, "Y"=1.0, "T"=2.0, "Enum"=enum."execute"}, {"X"=0.0, "Y"=1.0, "T"=2.0, "Enum"=enum."execute"}, {"X"=-1.0, "Y"=1.0, "T"=2.0, "Enum"=enum."execute"}, {"X"=0.0, "Y"=0.0, "T"=2.0, "Enum"=enum."wait"}] -> [w324] mode=indexing
          n122 = Enqueue Element(queue=w328, element=w324, error in (no error)=w327) -> (queue out=w325:refnum<queue>, error out=w326:errorcluster)  [unwired: 1 in, 1 out]
        }
      }
    }
    n123 = Wait Until Next ms Multiple(millisecond multiple=u32 20) -> ()  [unwired: 1 out]
  }
  n124 = String To IP(1:"localhost") -> (0:w16:u32)
  n125 = UDP Open(7:w16, 11:u16 1122 ("port")) -> (port=w15:refnum<k16>, 0:w14:errorcluster)  [unwired: 3 in, 1 out]
  n126 = call-poly <vilib>:"Add Object.vi"("New Object In"=w21, "Scene Object In"=w29) -> ("Scene Object Out"=w28:refnum<vi>)  [unwired: 8 in, 1 out]
  n127 = while {
    tunnel: w52 -> [w357]
    shift-right: [w356] -> w54
    shift-left: w28 -> [w356]
    shift-right: [w358] -> _
    shift-left: w53 -> [w358]
    tunnel: [w354] -> _
    stop <- w334 stop-if-true
    # "update the joint angles\nin the 3D representation"
    n128 = call <vilib>:"Update Joints.vi"("error in (no error)"=w357, "Joints"="Joint angles", "Joint Array"=w358) -> ("error out"=w355:errorcluster)  [unwired: 8 in]
    n129 = flat-sequence {
      tunnel: w356 -> [w360]
      tunnel: w355 -> [w359]
      tunnel: [w359] -> w354
      frame #0 {
        # "Display 3D representation"
        "3D robotic arm" <- w360
      }
    }
    n130 = Index Array(array="Joint angles requested", index=1) -> (element=w339:dbl)
    n131 = Index Array(array="Joint angles", index=1) -> (element=w343:dbl)
    n132 = Index Array(array="Joint angles requested", index=2) -> (element=w336:dbl)
    n133 = Index Array(array="Joint angles", index=2) -> (element=w338:dbl)
    n134 = expression code="(x/pi)*180.0" "radians to degrees"(w339) -> (w340:dbl)
    n135 = expression code="(x/pi)*180.0" "radians to degrees"(w343) -> (w342:dbl)
    n136 = expression code="(x/pi)*180.0" "radians to degrees"(w336) -> (w335:dbl)
    n137 = expression code="(x/pi)*180.0" "radians to degrees"(w338) -> (w337:dbl)
    n138 = Subtract(x=w340, y=w342) -> (x-y=→"error joint 1":dbl)
    n139 = Subtract(x=w335, y=w337) -> (x-y=→"error joint 2":dbl)
    n140 = Bundle("Joint Angles"=w342, "Joint Angles"=w340) -> (→"axis 1":cluster{"Joint Angles":dbl, "Joint Angles":dbl})  [unwired: 1 in]
    n141 = Bundle("Joint Angles"=w337, "Joint Angles"=w335) -> (→"axis 2":cluster{"Joint Angles":dbl, "Joint Angles":dbl})  [unwired: 1 in]
    n142 = Wait Until Next ms Multiple(millisecond multiple=u32 1) -> ()  [unwired: 1 out]
    n143 = local read "stop"() -> (w334:bool)
  }
  n144 = while {
    tunnel: w15 -> [w373]
    tunnel: w14 -> [w374]
    tunnel: [w367] -> w2
    tunnel: [w368] -> w3
    shift-right: [w365] -> w4
    shift-left: 0.0 -> [w364]
    shift-right: [w366] -> _
    shift-left: 0.0 -> [w363]
    tunnel: w1 -> [_]
    stop <- w361 stop-if-true
    n145 = UDP Read(connection ID=w373, max size (548)=1024, timeout ms (25000)=10, 8:w374) -> (data out=w370:string, error out=w371:errorcluster, 3:w368:refnum<k16>)  [unwired: 2 out]
    n146 = case shown="Error" w371 {
      selector: w371 -> [w379 w392]
      tunnel: w370 -> [w391 _]
      tunnel: [w379 w393] -> w367
      tunnel: [w375 w395] -> w366
      tunnel: [w376 w396] -> w365
      tunnel: w364 -> [_ w396]
      tunnel: w363 -> [_ w395]
      frame No Error {
        n147 = Match Pattern(string=w391, regular expression=",") -> (before substring=w389:string, after substring=w388:string)  [unwired: 1 in, 2 out]
        n148 = Match Pattern(string=w388, regular expression="\\]$") -> (before substring=w385:string)  [unwired: 1 in, 3 out]
        n149 = Match Pattern(string=w389, regular expression="^\\[") -> (after substring=w384:string)  [unwired: 1 in, 3 out]
        n150 = Fract/Exp String To Number(use system decimal point (T)=FALSE, string=w384, default (0 dbl)=0.0 ("default (0 DBL)")) -> (number=w377:dbl)  [unwired: 1 in, 1 out]
        n151 = Fract/Exp String To Number(use system decimal point (T)=FALSE, string=w385, default (0 dbl)=0.0 ("default (0 DBL)")) -> (number=w375:dbl)  [unwired: 1 in, 1 out]
        "UDP Y" <- w375
        "UDP Y" <- w375
        n152 = Multiply(x=w377, y=1.5) -> (x*y=w376:dbl)
        "UDP X" <- w376
        "UDP X" <- w376
      }
      frame Error {
        n153 = Unbundle By Name(w392) -> ("code"=w394:i32)
        n154 = case shown="56" w394 {
          tunnel: [w397 errorcluster {"status"=FALSE, "code"=0, "source"=""} ("error IO")] -> w393
          tunnel: w392 -> [w397 _]
          frame Default {
          }
          frame 56 {
          }
        }
      }
    }
    n155 = local read "stop"() -> (w361:bool)
    n156 = Wait Until Next ms Multiple(millisecond multiple=u32 1 ("milliseconds to wait")) -> ()  [unwired: 1 out]
  }
  n157 = while {
    tunnel: w25 -> [w412]
    shift-right: [w408] -> _
    shift-left: w24 -> [w411]
    shift-right: [w399] -> _
    shift-left: w23 -> [w406]
    shift-right: [w407] -> _
    shift-left: w23 -> [w405]
    tunnel: [w402] -> w11
    stop <- w413 stop-if-true
    n158 = call-poly <vilib>:"Acquire Input Data.vi"("device ID"=w412, "error in (no error)"=w411) -> ("device ID"=w402:refnum<k1>, "axis info"=w401:T27, "button info"=w403:T28, "error out"=w408:errorcluster)  [unwired: 13 in, 1 out]
    n159 = Wait Until Next ms Multiple(millisecond multiple=u32 20) -> ()  [unwired: 1 out]
    n160 = Unbundle By Name(w403) -> ()  [unwired: 4 out]
    n161 = Unbundle By Name(w401) -> ("X axis"=w400:i32, "Y axis"=w410:i32)  [unwired: 1 out]
    n162 = formula code="if(X>25000)\n{\nif(Xold<1.5)\n{\nXnew=Xold+step;\n}\n}\nif(X<-25000)\n{\n\nif(Xold>-1.5)\n{\nXnew=Xold-step;\n}\n}\nif(Y<-25000)\n{\nif(Yold<1)\n{\nYnew=Yold+step;\n}\n}\nif(Y>25000)\n{\nif(Yold>-1)\n{\nYnew=Yold-step;\n}\n}"("X"=w400, "Y"=w410, "step"=0.02 ("input variable"), "Xold"=w406, "Yold"=w405) -> ("Xnew"=w399:dbl, "Ynew"=w407:dbl)
    "Xcontroller" <- w399
    "Ycontroller" <- w407
    n163 = local read "stop"() -> (w413:bool)
  }
  n164 = Divide(x=w39, y=1000.0) -> (x/y=w40:dbl)
  n165 = node-c288(w39) -> (w48:T20)  [unwired: 3 in]
  n166 = timed-loop "Timed Loop" {
    shift-right: [w417] -> w50
    shift-left: T3 [[0.0], [0.0]] ("Q") -> [w420]
    shift-right: [w418] -> _
    shift-left: T3 [[0.0], [0.0]] ("Q") -> [w419]
    timing: w48 -> [_]
    timing-out: [_] -> w47
    tunnel: w42 -> [_]
    tunnel: w40 -> [w416]
    stop <- w433 stop-if-true
    (unwired) FALSE
    # "SIMULATION DIAGRAM"
    n167 = node-c288() -> ()  [unwired: 1 in, 1 out]
    n168 = local read "T"() -> (w421:T3)
    n169 = call "racunanje ddQ.vi"("T"=w421, "dQ"=w419, "g"=-9.8, "Q"=w420) -> ("ddQ"=w429:T3)  [unwired: 7 in]
    n170 = call-poly <vilib>:"Multiply.vi"("Real Matrix A"=w429, "Real Scalar c"=w416) -> ("c * A"=w430:T3)
    n171 = call-poly <vilib>:"Add.vi"("Real Matrix B"=w419, "Real Matrix A"=w430) -> ("A + B"=w418:T3)
    "dQ" <- w418
    n172 = call-poly <vilib>:"Multiply.vi"("Real Matrix A"=w418, "Real Scalar c"=w416) -> ("c * A"=w428:T3)
    n173 = call-poly <vilib>:"Add.vi"("Real Matrix B"=w428, "Real Matrix A"=w420) -> ("A + B"=w417:T3)
    "Q" <- w417
    n174 = Index Array(array=w417, index (row)=0, index (col)=0) -> (element=w415:dbl)
    n175 = Index Array(array=w417, index (row)=1, index (col)=0) -> (element=w414:dbl)
    n176 = Build Array(3.14 ("element"), w415, w414, 0.0 ("element")) -> (w427:dbl[])
    n177 = local write "Joint angles"(w427) -> ()
    n178 = local read "stop"() -> (w433:bool)
    n179 = node-c288() -> ()  [unwired: 1 in, 1 out]
  }
  n180 = node-c288(w47) -> ()  [unwired: 1 out]
  n181 = node-c288(w45) -> ()  [unwired: 1 out]
  n182 = flat-sequence {
    tunnel: w54 -> [w441]
    tunnel: w50 -> [_]
    tunnel: w5 -> [w440]
    tunnel: w11 -> [w439]
    tunnel: w10 -> [_]
    tunnel: w4 -> [_]
    tunnel: w3 -> [w437]
    tunnel: w2 -> [w436]
    frame #0 {
      n183 = UDP Close(connection ID=w437, 8:w436) -> (error out=w438:errorcluster)  [unwired: 1 out]
      n184 = Flush Queue(queue=w440) -> ()  [unwired: 1 in, 3 out]
      n185 = Close Reference(reference=w441) -> ()  [unwired: 1 in, 1 out]
      n186 = call-poly <vilib>:"Close Input Device.vi"("device ID"=w439) -> ()  [unwired: 9 in, 1 out]
      n187 = call <vilib>:"Simple Error Handler.vi"("error in (no error)"=w438) -> ()  [unwired: 4 in, 5 out]
    }
  }
